vi "Toggle8.vi"(8 "error in":errorcluster, 11 "RawInput":bool) -> (0 "error out":errorcluster, 3 "ToggleState":bool)   [LabVIEW 2013]
doc: "General-purpose VI for handling toggle input. RawInput is the raw value of the button, and ToggleState is whether that button is currently toggled or not. ToggleState starts out as false, and every time the button is pressed, ToggleState changes state."
uses:
  Robot_Framework_2014/ToggleAction.ctl
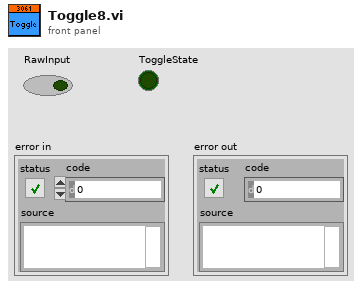
[diagram p1: front panel]
types:
  T1 = typedef "ToggleAction.ctl" = enum16{"Retract2", "Actuate1", "Actuate2", "Retract1"}
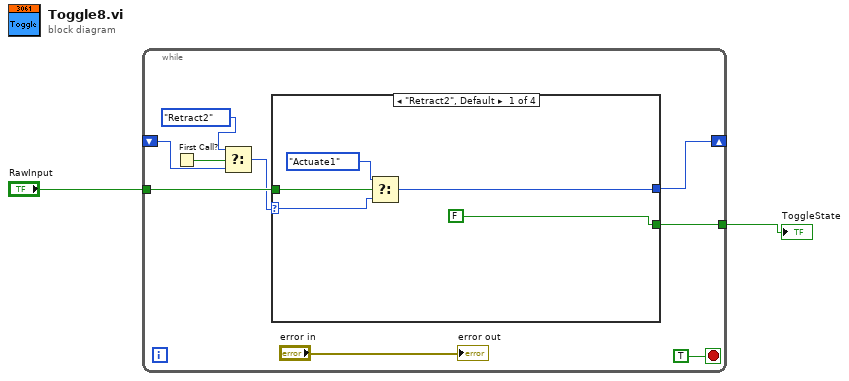
[diagram p0: block diagram]
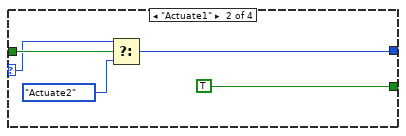
[diagram p2: hidden frame]
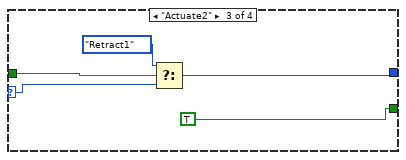
[diagram p3: hidden frame]
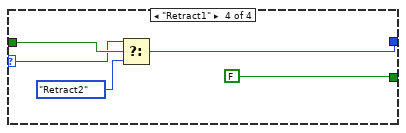
[diagram p4: hidden frame]
diagram:
  n1 = while {
    tunnel: "RawInput" -> [w10]
    shift-right: [w9] -> _
    shift-left: _ -> [w6]
    tunnel: [w8] -> w1
    stop <- TRUE stop-if-true
    n2 = First Call?() -> (First Call?: T/F=w7:bool)
    n3 = Select(t=ToggleAction."Retract2" ("Enum"), s=w7, f=w6) -> (s? t:f=w4:T1)
    n4 = case shown="\"Retract2\", Default" w4 {
      selector: w4 -> [w15 w17 w22 w27]
      tunnel: w10 -> [w16 w21 w26 w30]
      tunnel: [w13 w19 w23 w29] -> w9
      tunnel: [FALSE TRUE TRUE FALSE] -> w8
      frame "Retract2", Default {
        n5 = Select(t=ToggleAction."Actuate1" ("Enum"), s=w16, f=w15) -> (s? t:f=w13:T1)
      }
      frame "Actuate1" {
        n6 = Select(t=w17, s=w21, f=ToggleAction."Actuate2" ("Enum")) -> (s? t:f=w19:T1)
      }
      frame "Actuate2" {
        n7 = Select(t=ToggleAction."Retract1" ("Enum"), s=w26, f=w22) -> (s? t:f=w23:T1)
      }
      frame "Retract1" {
        n8 = Select(t=w27, s=w30, f=ToggleAction."Retract2" ("t")) -> (s? t:f=w29:T1)
      }
    }
    "error out" <- "error in"
  }
  "ToggleState" <- w1
